vi "SwerveKinematics_NewX.vi"(11 "Wheels":T1[](array[typedef]) {"Y" format="%14.3f"; "X" format="%14.3f"}) -> (3 "SWERVE_DRIVE_KINEMATICS":T2 {"SavedModuleStates"."Angle"."SIN" format="%13.4f"; "SavedModuleStates"."Angle"."COS" format="%13.4f"; "SavedModuleStates"."Angle"."VALUE" format="%13.4f"; "PrevCoR"."Y" format="%14.3f"; "PrevCoR"."X" format="%14.3f"; "Modules"."Y" format="%14.3f"; "Modules"."X" format="%14.3f"})   [LabVIEW 2019, in "Trajectory_Library.lvlib"]
doc: "Constructs a swerve drive kinematics object. This takes in a variable number of wheel locations as Translation2ds. The order in which you pass in the wheel locations is the same order that you will recieve the module states when performing inverse kinematics. It is also expected that you pass in the module states in the same order when calling the forward kinematics methods.\n\nThis is a helper class that converts a chassis velocity (dx, dy, and dtheta components) into individual module states (speed and angle).\n \nThe inverse kinematics (converting from a desired chassis velocity to individual module states) uses the relative locations of the modules with respect to the center of rotation. The center of rotation for inverse kinematics is also variable. This means that you can set your set your center of rotation in a corner of the robot to perform special evasion manuevers.\n \nForward kinematics (converting an array of module states into the overall chassis motion) is performs the exact opposite of what inverse kinematics does. Since this is an overdetermined system (more equations than variables), we use a least-squares approximation.\n \nThe inverse kinematics: [moduleStates] = [moduleLocations][chassisSpeeds] We take the Moore-Penrose pseudoinverse of [moduleLocations] and then multiply by [moduleStates] to get our chassis speeds.\n \nForward kinematics is also used for odometry -- determining the position of the robot on the field using encoders and a gyro.\n\nParameters: \n - wheels - Array of Translation data structures indicating the locations of the wheels relative to the physical center of the robot. (Meters)\n\nReturns:\n - SwerveDriveKinematics - The initialized data structure"
uses:
  Trajectory_Library.lvlib
  <vilib>/Analysis/Matrix/Datatypes/RealMatrix.ctl
  <vilib>/Analysis/Matrix/NI_Matrix.lvlib
  TypeDef/TRANSLATION2D.ctl
  TypeDef/SWERVE_DRIVE_KINEMATICS.ctl
  <vilib>/Analysis/NI_AALPro.lvlib
  <vilib>/Analysis/_algsub.llb/Real PseudoInverse Matrix.vi
  <vilib>/Rock Robotics/SystemInterfaces/NetworkCommunication/NetComm_UsageReport_ResourceType.ctl
  Util_LibraryGlobals.vi
  TypeDef/ROTATION2D.ctl
  TypeDef/SWERVE_DRIVE_MODULE_STATE.ctl
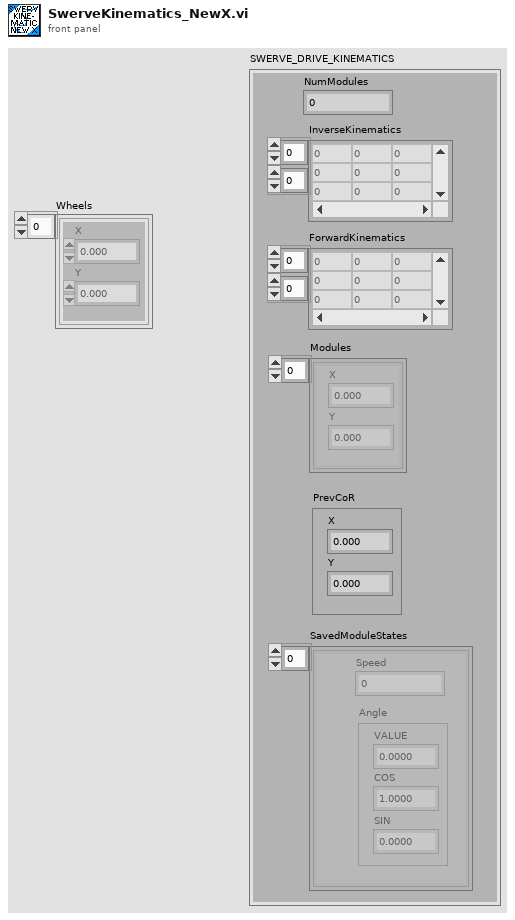
[diagram p1: front panel]
types:
  T1 = typedef "Trajectory_Library.lvlib/TRANSLATION2D.ctl" = cluster{"X":dbl, "Y":dbl}
  T2 = typedef "Trajectory_Library.lvlib/SWERVE_DRIVE_KINEMATICS.ctl" = cluster{"NumModules":i32, "InverseKinematics":T3, "ForwardKinematics":T3, "Modules":T1[], "PrevCoR":T1, "SavedModuleStates":T4[]}
  T3 = typedef "NI_Matrix.lvlib/RealMatrix.ctl" = dbl[][]
  T4 = typedef "Trajectory_Library.lvlib/SWERVE_DRIVE_MODULE_STATE.ctl" = cluster{"Speed":dbl, "Angle":T5}
  T5 = typedef "Trajectory_Library.lvlib/ROTATION2D.ctl" = cluster{"VALUE":dbl, "COS":dbl, "SIN":dbl}
  T6 = typedef "NetComm_UsageReport_ResourceType.ctl" = enum8{"Controller", "Module", "Language", "CANPlugin", "Accelerometer", "ADXL345", "AnalogChannel", "AnalogTrigger", "AnalogTriggerOutput", "CANJaguar", "Compressor", "Counter", "Dashboard", "DigitalInput", "DigitalOutput", "DriverStationCIO", "DriverStationEIO", "DriverStationLCD", "Encoder", "GearTooth", "Gyro", "I2C", "Framework", "Jaguar", "Joystick", "Kinect", "KinectStick", "PIDController", "Preferences", "PWM", "Relay", "RobotDrive", "SerialPort", "Servo", "Solenoid", "SPI", "Task", "Ultrasonic", "Victor", "Button", "Command", "AxisCamera", "PCVideoServer", "SmartDashboard", "Talon", "HiTechnicColorSensor", "HiTechnicAccel", "HiTechnicCompass", "SRF08", "AnalogOutput", "Victor SP", "Talon SRX", "CAN Talon SRX", "ADXL362 Accel", "ADXRS450 Gyro", "Rev SPARK", "Mindsensors SD540", "Digital Filter", "ADIS16448", "PDP", "PCM", "PigeonIMU", "Nidec Brushless", "CTRE CANifier", "CTRE TalonFX", "CTRE Future 1", "CTRE Future 2", "CTRE Future 3", "CTRE Future 4", "CTRE Future 5", "CTRE Future 6", "Linear Filter", "Xbox Controller", "USB Camera", "NavX", "Pixy", "Pixy2", "ScanseSweep", "Shuffleboard", "CAN", "Digilent DMC60", "PWM Victor SPX", "Rev SPARK MAX PWM", "Rev SPARK MAX CAN", "ADIS16470", "PIDController2", "ProfiledPIDController", "Kinematics", "Odometry", "Units", "Trapezoid Profile", "DutyCycle", "Addressable LEDs", "Fusion Venom"}
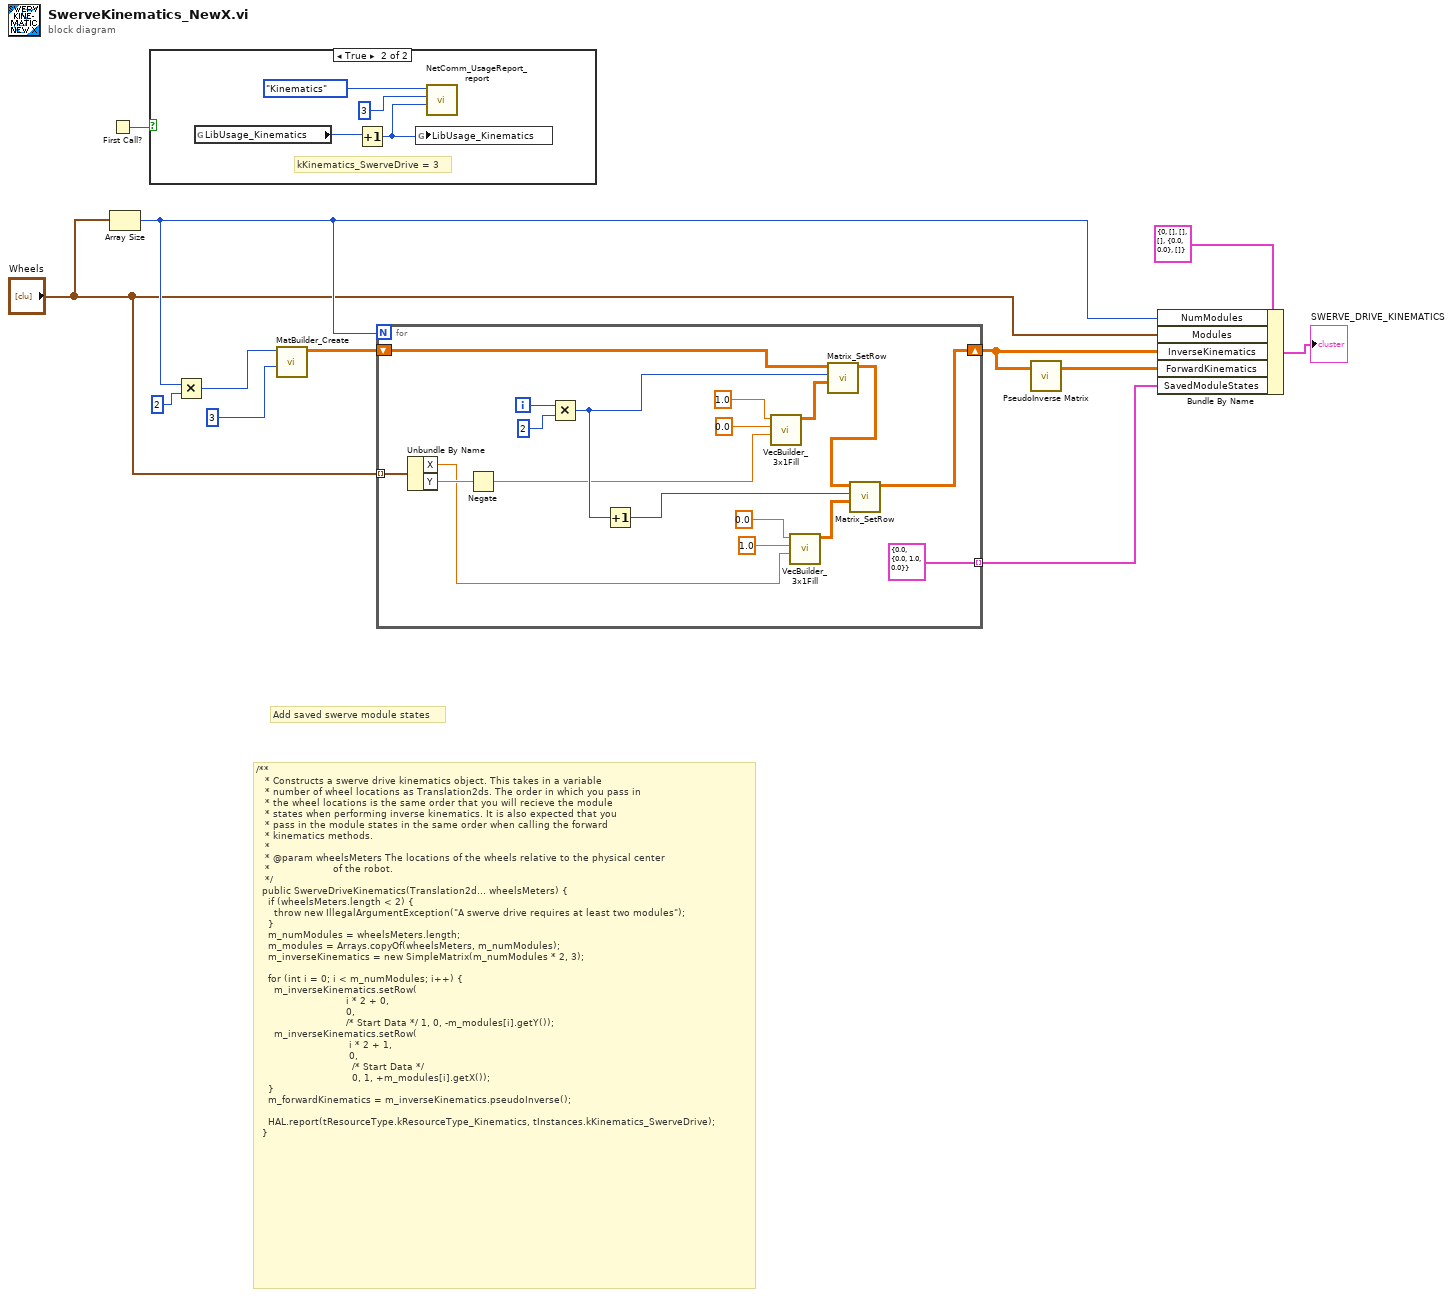
[diagram p0: block diagram]
diagram:
  # "Add saved swerve module states"
  # "/**\n   * Constructs a swerve drive kinematics object. This takes in a variable\n   * number of wheel locations as Translation2ds. The order in which you pass in\n   * the wheel locations is the same order that you will recieve the module\n   * states when performing inverse kinematics. It is also expected that you\n   * pass in the module states in the same order when calling the forward\n   * kinematics methods.\n   *\n   * @param wheelsMeters The locations of the wheels relative to the physical center\n   *                     of the robot.\n   */\n  public SwerveDriveKinematics(Translation2d... wheelsMeters) {\n    if (wheelsMeters.length < 2) {\n      throw new IllegalArgumentException(\"A swerve drive requires at least two modules\");\n    }\n    m_numModules = wheelsMeters.length;\n    m_modules = Arrays.copyOf(wheelsMeters, m_numModules);\n    m_inverseKinematics = new SimpleMatrix(m_numModules * 2, 3);\n\n    for (int i = 0; i < m_numModules; i++) {\n      m_inverseKinematics.setRow(\n                              i * 2 + 0, \n                              0, \n                              /* Start Data */ 1, 0, -m_modules[i].getY());\n      m_inverseKinematics.setRow(\n                               i * 2 + 1, \n                               0, \n                                /* Start Data */ \n                                0, 1, +m_modules[i].getX());\n    }\n    m_forwardKinematics = m_inverseKinematics.pseudoInverse();\n\n    HAL.report(tResourceType.kResourceType_Kinematics, tInstances.kKinematics_SwerveDrive);\n  }"
  n1 = First Call?() -> (First Call?: T/F=w5:bool)
  n2 = Array Size(array="Wheels") -> (size(s)=w8:i32)
  n3 = case shown="True" w5 {
    frame False {
    }
    frame True {
      # "kKinematics_SwerveDrive = 3"
      n4 = global read "Util_LibraryGlobals.vi" "LibUsage_Kinematics"() -> (w15:i32)
      n5 = Increment(x=w15) -> (x+1=w14:i32)
      n6 = global write "Util_LibraryGlobals.vi" "LibUsage_Kinematics"(w14) -> ()
      n7 = call <vilib>:"NetComm_UsageReport_report.vi"("Context"=w14, "Instance Number"=u8 3, "Resource Type"=NetComm_UsageReport_ResourceType."Kinematics") -> ()  [unwired: 9 in]
    }
  }
  n8 = Multiply(x=w8, y=2) -> (x*y=w4:i32)
  n9 = call "MatBuilder_Create.vi"("Columns"=3 ("number of columns"), "Rows"=w4) -> ("output matrix"=w2:T3)  [unwired: 9 in]
  n10 = for {
    N: w8 -> [_]
    shift-right: [w22] -> w6
    shift-left: w2 -> [w24]
    tunnel: "Wheels" -> [w32] mode=indexing
    tunnel: [T4 {"Speed"=0.0, "Angle"={"VALUE"=0.0, "COS"=1.0, "SIN"=0.0}} ("SWERVE_DRIVE_MODULE_STATE")] -> w1 mode=indexing
    i -> [w34]
    n11 = Unbundle By Name(w32) -> ("X"=w18:dbl, "Y"=w31:dbl)
    n12 = Negate(x=w31) -> (-x=w19:dbl)
    n13 = Multiply(x=w34, y=2) -> (x*y=w21:i32)
    n14 = Increment(x=w21) -> (x+1=w20:i32)
    n15 = call "VecBuilder_3x1Fill.vi"("R2"=w19, "R1"=0.0, "R0"=1.0) -> ("output matrix"=w29:T3)  [unwired: 8 in]
    n16 = call "VecBuilder_3x1Fill.vi"("R2"=w18, "R1"=1.0, "R0"=0.0) -> ("output matrix"=w30:T3)  [unwired: 8 in]
    n17 = call "Matrix_SetRow.vi"("Fill Row Vector"=w29, "Row"=w21, "input matrix"=w24) -> ("output matrix"=w23:T3)  [unwired: 7 in, 1 out]
    n18 = call "Matrix_SetRow.vi"("Fill Row Vector"=w30, "Row"=w20, "input matrix"=w23) -> ("output matrix"=w22:T3)  [unwired: 7 in, 1 out]
  }
  n19 = call-poly <vilib>:"PseudoInverse Matrix.vi"("Input Matrix"=w6) -> ("PseudoInverse Matrix"=w9:T3)  [unwired: 1 in, 1 out]
  n20 = Bundle By Name(cluster=T2 {"NumModules"=0, "InverseKinematics"=[], "ForwardKinematics"=[], "Modules"=[], "PrevCoR"={"X"=0.0, "Y"=0.0}, "SavedModuleStates"=[]} ("SWERVE_DRIVE_KINEMATICS"), "NumModules"=w8, "Modules"="Wheels", "InverseKinematics"=w6, "ForwardKinematics"=w9, "SavedModuleStates"=w1) -> (→"SWERVE_DRIVE_KINEMATICS":T2)
